vi "Ini2Array.vi"(2 "error in (no error)":errorcluster caption="错误输入（无错误）", 3 "路径":path) -> (0 "error out":errorcluster caption="错误输出", 1 "数组":T1[](array[typedef]))   [LabVIEW 2019]
uses:
  ctl/InfoOfPlayer.ctl
  <vilib>/Utility/config.llb/NI_LVConfig.lvlib
panel:
  in  "玩家信息":T1
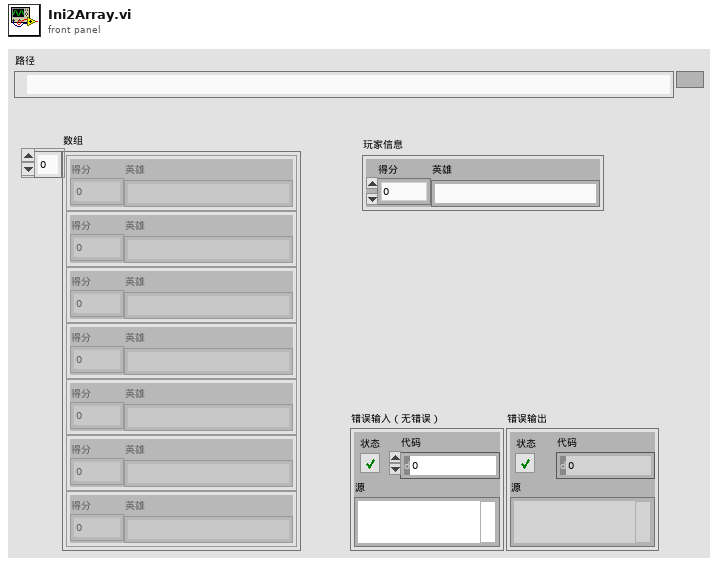
[diagram p1: front panel]
types:
  T1 = typedef "InfoOfPlayer.ctl" = cluster{"得分":i32, "英雄":string}
  T2 = typedef "NI_LVConfig.lvlib/Config Data RefNum.ctl" = refnum<k1>
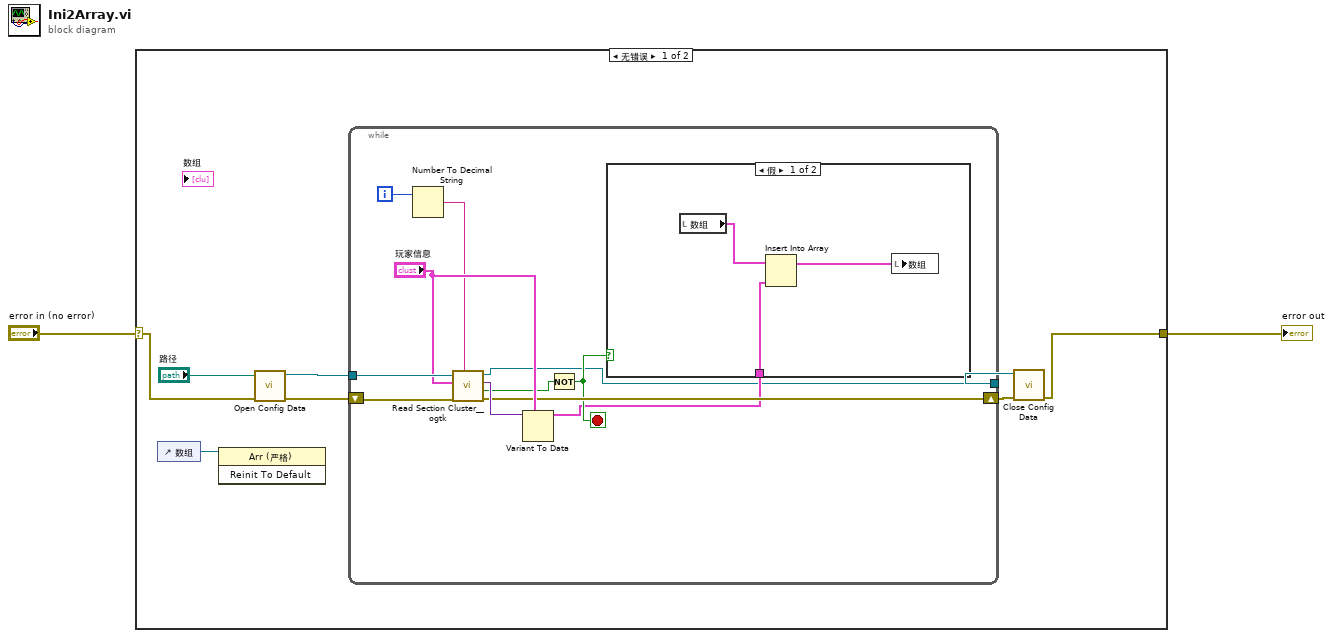
[diagram p0: block diagram]
diagram:
  n1 = case shown="无错误" "error in (no error)" {
    selector: "error in (no error)" -> [w5 w25]
    tunnel: [w4 w25] -> w1
    frame No Error {
      n2 = control-ref of="数组"() -> (w3:refnum<vi>)
      n3 = invoke class="Arr (严格)" method="Reinit To Default"(reference=w3) -> ()  [unwired: 2 in, 3 out]
      n4 = call <vilib>:"Open Config Data.vi"("error in (no error)"=w5, "configuration file path"="路径") -> ("error out"=w8:errorcluster, "refnum"=w9:T2)  [unwired: 7 in, 1 out]
      n5 = while {
        tunnel: w9 -> [w21]
        shift-right: [w17] -> w7
        shift-left: w8 -> [w18]
        tunnel: [w11] -> w6
        i -> [w16]
        stop <- w13 stop-if-true
        n6 = Number To Decimal String(number=w16) -> (decimal integer string=w15:string)  [unwired: 1 in]
        n7 = call <userlib>:"Read Section Cluster__ogtk.vi"("section (optional)"=w15, "error in (no error)"=w18, "Section Formatted Cluster Type"="玩家信息", "refnum"=w21) -> ("error out"=w17:errorcluster, "all found?"=w14:bool, "Section Formatted Cluster"=w20:variant, "dup refnum"=w11:T2)  [unwired: 3 in, 1 out]
        n8 = Variant To Data(type="玩家信息", Variant=w20) -> (data=w12:T1)  [unwired: 1 in, 1 out]
        n9 = Not(x=w14) -> (.not. x?=w13:bool)
        n10 = case shown="假" w13 {
          tunnel: w12 -> [w22 _]
          frame False {
            n11 = local read "数组"() -> (w24:T1[])
            n12 = Insert Into Array(array=w24, new element=w22) -> (w23:T1[])  [unwired: 1 in]
            n13 = local write "数组"(w23) -> ()
          }
          frame True {
          }
        }
      }
      n14 = call <vilib>:"Close Config Data.vi"("error in (no error)"=w7, "refnum"=w6) -> ("error out"=w4:errorcluster)  [unwired: 8 in, 1 out]
    }
    frame Error {
    }
  }
  "error out" <- w1
